vi "例程11-全局变量的使用.vi"() -> ()   [LabVIEW 2016]
panel:
  out "数值":i32
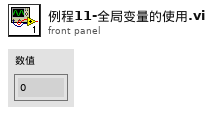
[diagram p1: front panel]
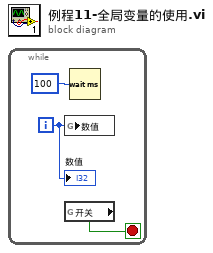
[diagram p0: block diagram]
diagram:
  n1 = while {
    i -> [w1]
    stop <- w2 stop-if-true
    n2 = global write "例程11-全局.vi" "数值"(w1) -> ()
    n3 = global read "例程11-全局.vi" "开关"() -> (w2:bool)
    n4 = Wait (ms)(milliseconds to wait=u32 100 ("等待时间（毫秒）")) -> ()  [unwired: 1 out]
    "数值" <- w1
  }
